vi "WLAN - Test - UTIL - GetTime.vi"(8 "error in (no error)":errorcluster) -> (0 "error out":errorcluster, 1 "millisecond timer value":u32, 4 "Tick Count(s)":dbl)   [LabVIEW 2011]
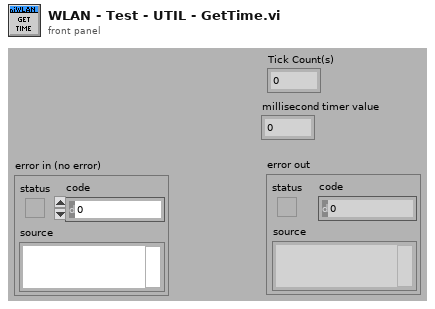
[diagram p1: front panel]
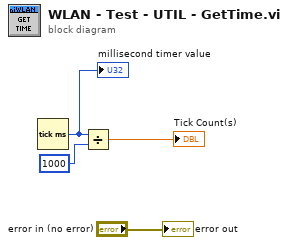
[diagram p0: block diagram]
diagram:
  n1 = Tick Count (ms)() -> (millisecond timer value=w3:u32)
  "millisecond timer value" <- w3
  n2 = Divide(x=w3, y=u32 1000) -> (x/y=→"Tick Count(s)":dbl)
  "error out" <- "error in (no error)"
